vi "apply seq channel changes.vi"(7 "owner ID":string, 8 "error in":errorcluster, 9 "modified seq channel":refnum<class "tag descriptor.lvclass">, 10 "original seq channel":refnum<class "tag descriptor.lvclass">, 11 "engine configuration in":refnum<class "base TBM sequencer configuration.lvclass">) -> (0 "error out":errorcluster, 3 "engine configuration out":refnum<class "base TBM sequencer configuration.lvclass">)   [LabVIEW 2014, in "base TBM sequencer configuration.lvclass"]
uses:
  base TBM sequencer configuration.lvclass
  <vilib>/NI/Tag Bus/tag/tag descriptor.lvclass
  <vilib>/NI/Tag Bus/tag/tag descriptor.lvclass/tag descriptor.ctl
  <vilib>/NI/Tag Bus/tag/read tag name.vi
  <vilib>/NI/Tag Bus/tag/read data type.vi
  <vilib>/NI/Tag Bus/tag/read metadata.vi
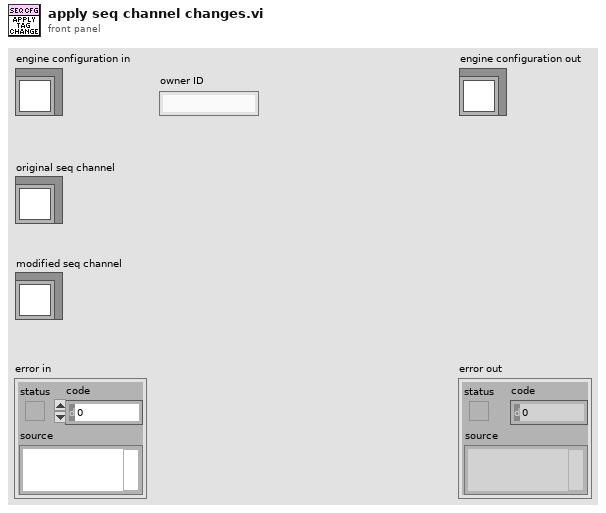
[diagram p1: front panel]
types:
  T1 = typedef "tag bus.lvlib/tag descriptor.lvclass/Data Type.ctl" = enum16{"Double", "Single", "I64", "I32", "I16", "I8", "U64", "U32", "U16", "U8", "Boolean", "String", "Array of Double", "Array of Single", "Array of I64", "Array of I32", "Array of I16", "Array of I8", "Array of U64", "Array of U32", "Array of U16", "Array of U8", "Array of Boolean", "Array of String"}
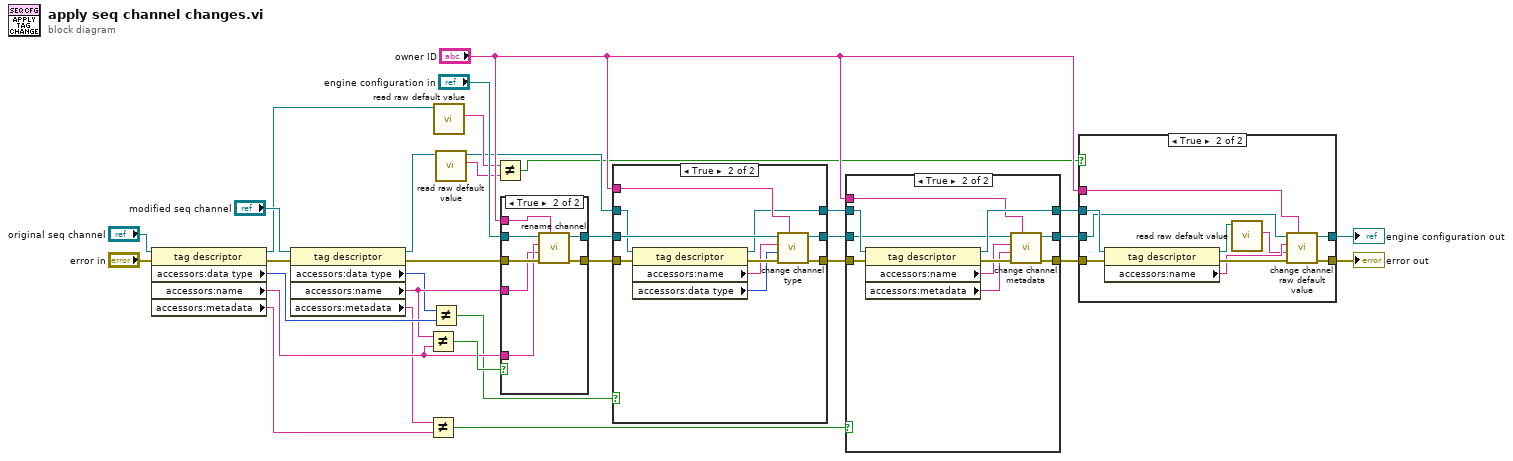
[diagram p0: block diagram]
diagram:
  n1 = property class="tag descriptor"(reference="original seq channel", error in="error in") -> (reference out=w6:refnum<class "tag descriptor.lvclass">, error out=w31:errorcluster, "accessors:data type"=w27:T1, "accessors:name"=w24:string, "accessors:metadata"=w16:string)
  n2 = property class="tag descriptor"(reference="modified seq channel", error in=w31) -> (reference out=w3:refnum<class "tag descriptor.lvclass">, error out=w26:errorcluster, "accessors:data type"=w19:T1, "accessors:name"=w20:string, "accessors:metadata"=w15:string)
  n3 = Not Equal?(x=w20, y=w24) -> (x != y?=w28:bool)
  n4 = Not Equal?(x=w15, y=w16) -> (x != y?=w14:bool)
  n5 = Not Equal?(x=w19, y=w27) -> (x != y?=w21:bool)
  n6 = call <vilib>:"read raw default value.vi"("system tag in"=w6) -> ("raw default"=w4:string)  [unwired: 8 in, 2 out]
  n7 = call <vilib>:"read raw default value.vi"("system tag in"=w3) -> ("raw default"=w5:string, "system tag out"=w2:refnum<class "tag descriptor.lvclass">)  [unwired: 8 in, 1 out]
  n8 = Not Equal?(x=w4, y=w5) -> (x != y?=w1:bool)
  n9 = case shown="True" w28 {
    tunnel: w26 -> [w33 w41]
    tunnel: "engine configuration in" -> [w34 w40]
    tunnel: [w34 w39] -> w22
    tunnel: "owner ID" -> [_ w38]
    tunnel: w24 -> [_ w37]
    tunnel: w20 -> [_ w36]
    tunnel: [w33 w35] -> w23
    frame False {
    }
    frame True {
      n10 = call "rename channel.vi"("owner ID"=w38, "error in"=w41, "new name"=w36, "old name"=w37, "engine configuration in"=w40) -> ("error out"=w35:errorcluster, "engine configuration out"=w39:refnum<class "base TBM sequencer configuration.lvclass">)  [unwired: 5 in]
    }
  }
  n11 = case shown="True" w21 {
    tunnel: w23 -> [w43 w50]
    tunnel: w22 -> [w44 w54]
    tunnel: [w44 w53] -> w18
    tunnel: "owner ID" -> [_ w51]
    tunnel: [w43 w52] -> w17
    tunnel: w2 -> [w42 w46]
    tunnel: [w42 w45] -> w13
    frame False {
    }
    frame True {
      n12 = property class="tag descriptor"(reference=w46, error in=w50) -> (reference out=w45:refnum<class "tag descriptor.lvclass">, error out=w49:errorcluster, "accessors:name"=w47:string, "accessors:data type"=w48:T1)
      n13 = call "change channel type.vi"("owner ID"=w51, "error in"=w49, "new data type"=w48, "channel name"=w47, "engine configuration in"=w54) -> ("error out"=w52:errorcluster, "engine configuration out"=w53:refnum<class "base TBM sequencer configuration.lvclass">)  [unwired: 5 in]
    }
  }
  n14 = case shown="True" w14 {
    tunnel: w17 -> [w56 w67]
    tunnel: w18 -> [w57 w58]
    tunnel: [w57 w63] -> w11
    tunnel: "owner ID" -> [_ w64]
    tunnel: [w56 w62] -> w12
    tunnel: w13 -> [w55 w66]
    tunnel: [w55 w65] -> w8
    frame False {
    }
    frame True {
      n15 = property class="tag descriptor"(reference=w66, error in=w67) -> (reference out=w65:refnum<class "tag descriptor.lvclass">, error out=w61:errorcluster, "accessors:name"=w59:string, "accessors:metadata"=w60:string)
      n16 = call "change channel metadata.vi"("owner ID"=w64, "error in"=w61, "metadata"=w60, "channel name"=w59, "engine configuration in"=w58) -> ("error out"=w62:errorcluster, "engine configuration out"=w63:refnum<class "base TBM sequencer configuration.lvclass">)  [unwired: 5 in]
    }
  }
  n17 = case shown="True" w1 {
    tunnel: w12 -> [w68 w79]
    tunnel: w11 -> [w69 w73]
    tunnel: [w69 w76] -> w10
    tunnel: "owner ID" -> [_ w72]
    tunnel: [w68 w75] -> w9
    tunnel: w8 -> [_ w78]
    frame False {
    }
    frame True {
      n18 = property class="tag descriptor"(reference=w78, error in=w79) -> (reference out=w77:refnum<class "tag descriptor.lvclass">, error out=w74:errorcluster, "accessors:name"=w71:string)
      n19 = call <vilib>:"read raw default value.vi"("system tag in"=w77) -> ("raw default"=w70:string)  [unwired: 8 in, 2 out]
      n20 = call "change channel raw default value.vi"("owner ID"=w72, "error in"=w74, "raw default"=w70, "channel name"=w71, "engine configuration in"=w73) -> ("error out"=w75:errorcluster, "engine configuration out"=w76:refnum<class "base TBM sequencer configuration.lvclass">)  [unwired: 5 in]
    }
  }
  "error out" <- w9
  "engine configuration out" <- w10
